vi "GetAliasState.vi"(0 "reference in":refnum<class "SwitchBase.lvclass">, 5 "error in (no error)":errorcluster) -> (14 "reference in":refnum<class "SwitchBase.lvclass">, 15 "Active":string, 17 "State":bool, 19 "error out":errorcluster)   [LabVIEW 2017]
uses:
  SwitchBase.lvclass
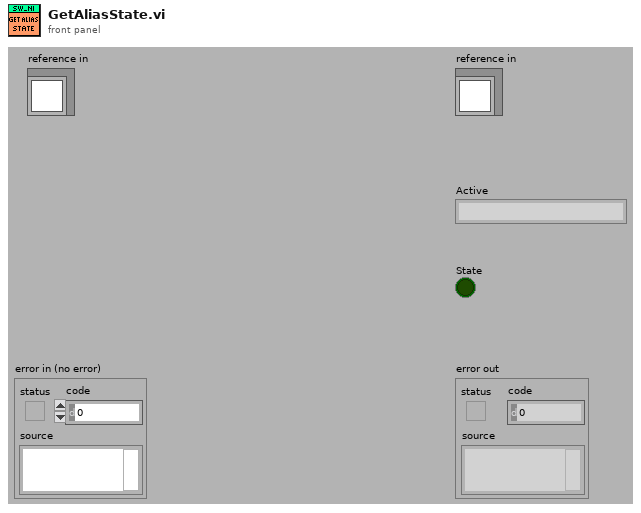
[diagram p1: front panel]
types:
  T1 = typedef "SwitchBase.lvlib/SwitchBase.lvclass/ObjectAttributes.ctl" = cluster{"Config":T2, "History":string[], "channel 1":string, "channel 2":string, "ActiveAlias":string, "AliasState":bool}
  T2 = typedef "SwitchBase.lvlib/SwitchBase.lvclass/Config.ctl" = cluster{"Resource":refnum<k15>, "topology name":T3, "Alias":cluster{"Name":string, "C1,C2":string[][]}[]}
  T3 = typedef "niSwitch Topologies.ctl" = string
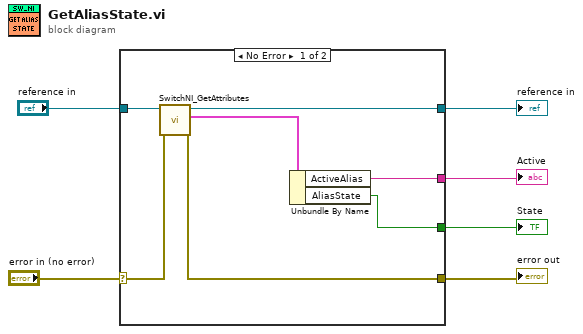
[diagram p0: block diagram]
diagram:
  n1 = case shown="No Error" "error in (no error)" {
    selector: "error in (no error)" -> [w13 w15]
    tunnel: [w11 w15] -> w5
    tunnel: [w9 w14] -> w3
    tunnel: "reference in" -> [w10 w14]
    tunnel: [w8 _] -> w2
    tunnel: [w7 _] -> w1
    frame No Error {
      n2 = call "SwitchNI_GetAttributes.vi"("error in (no error)"=w13, "reference in"=w10) -> ("error out"=w11:errorcluster, "Data"=w12:T1, "reference out"=w9:refnum<class "SwitchBase.lvclass">)  [unwired: 6 in, 1 out]
      n3 = Unbundle By Name(w12) -> ("ActiveAlias"=w8:string, "AliasState"=w7:bool)
    }
    frame Error {
    }
  }
  "error out" <- w5
  "reference in" <- w3
  "Active" <- w2
  "State" <- w1
